vi "Controller server w pressure control.vi"() -> ()   [LabVIEW 2017]
uses:
  <vilib>/DAQmx/write.llb/DAQmx Write (Digital Bool 1Line 1Point).vi
  <vilib>/DAQmx/write.llb/DAQmx Write (Digital 1D Bool NChan 1Samp 1Line).vi
  <vilib>/DAQmx/read.llb/DAQmx Read (Digital 1D Bool NChan 1Samp 1Line).vi
  <vilib>/DAQmx/miscellaneous.llb/DAQmx Fill In Error Info.vi
panel:
  in  "Switch time (s)":dbl=20.0
  in  "Switch polarity":bool
  in  "Pressure control (psi)":dbl=40.0
  out "Gauge Pressure (psi)":dbl
  in  "Pressure controller":T1={"Unit ID"="A", "Baud Rate"=enum."19200", "VISA Sesssion In"="COM8"}
  in  "Potentiostat power":bool
  out "ALS START":bool
  in  "ALS START Contr.":bool
  in  "Valve 4 Contr.":bool
  out "HPLC pressure voltage":dbl format="%0.3f"
  out "ALS Ready":bool
  out "Valve 4":bool
  out "Pressure 2 (psi)":dbl
  in  "Pressure 2 calibrate":bool
  in  "50 psi voltage":dbl=1.184
  in  "200 psi voltage":dbl=3.211
  out "Pressure 2 voltage":dbl format="%0.3f"
  in  "A 3":dbl=74.00098667982239
  in  "B 3":dbl=-37.617168228909705
  out "Pressure 1 (psi)":dbl
  out "Pressure 1 voltage":dbl format="%0.3f"
  in  "Pressure 1 calibrate":bool
  in  "10 psi voltage":dbl=1.224
  in  "130 psi voltage":dbl=4.215
  in  "B 2":dbl=-39.1073219658977
  in  "A 2":dbl=40.120361083249755
  in  "0ml voltage":dbl=1.137
  in  "6ml voltage":dbl=3.445
  out "Position voltage":dbl format="%0.3f"
  in  "B 2":dbl=-2.9558058925476605
  in  "A 1":dbl=2.5996533795493937
  in  "Position calibrate":bool
  out "Pump 1 position":dbl format="%0.2f"
  in  "stop":bool
  in  "Manual control":bool
  out "HPLC pressure (bar)":dbl(graph)
  in  "Phase sensor calibrate":bool[](array[boolean])
  out "Phase sensor analog 6":dbl(graph)
  out "Phase sensor analog 5":dbl(graph)
  out "Valve 3":bool
  out "Valve 1 position":i32 max=1
  in  "Valve 3 Contr.":bool
  in  "Valve 2 Contr.":bool
  in  "Valve 1 Contr.":bool
  in  "HPLC SHUT DOWN Contr.":bool
  in  "HPLC START REQUEST Contr.":bool
  in  "HPLC STOP Contr.":bool
  in  "HPLC START Contr.":bool
  out "HPLC Ready":bool
  out "HPLC START REQUEST":bool
  out "HPLC STOP":bool
  out "HPLC SHUT DOWN":bool
  out "HPLC START":bool
  out "Phase sensor digital":bool[](array[boolean])
  out "Valve 1":bool
  out "Valve 2":bool
  out "Phase sensor analog 1":dbl(graph)
  out "Phase sensor analog 2":dbl(graph)
  out "Phase sensor analog 3":dbl(graph)
  out "Phase sensor analog 4":dbl(graph)
  # "Pressure transducer 1"
  # "Pressure transducer 2"
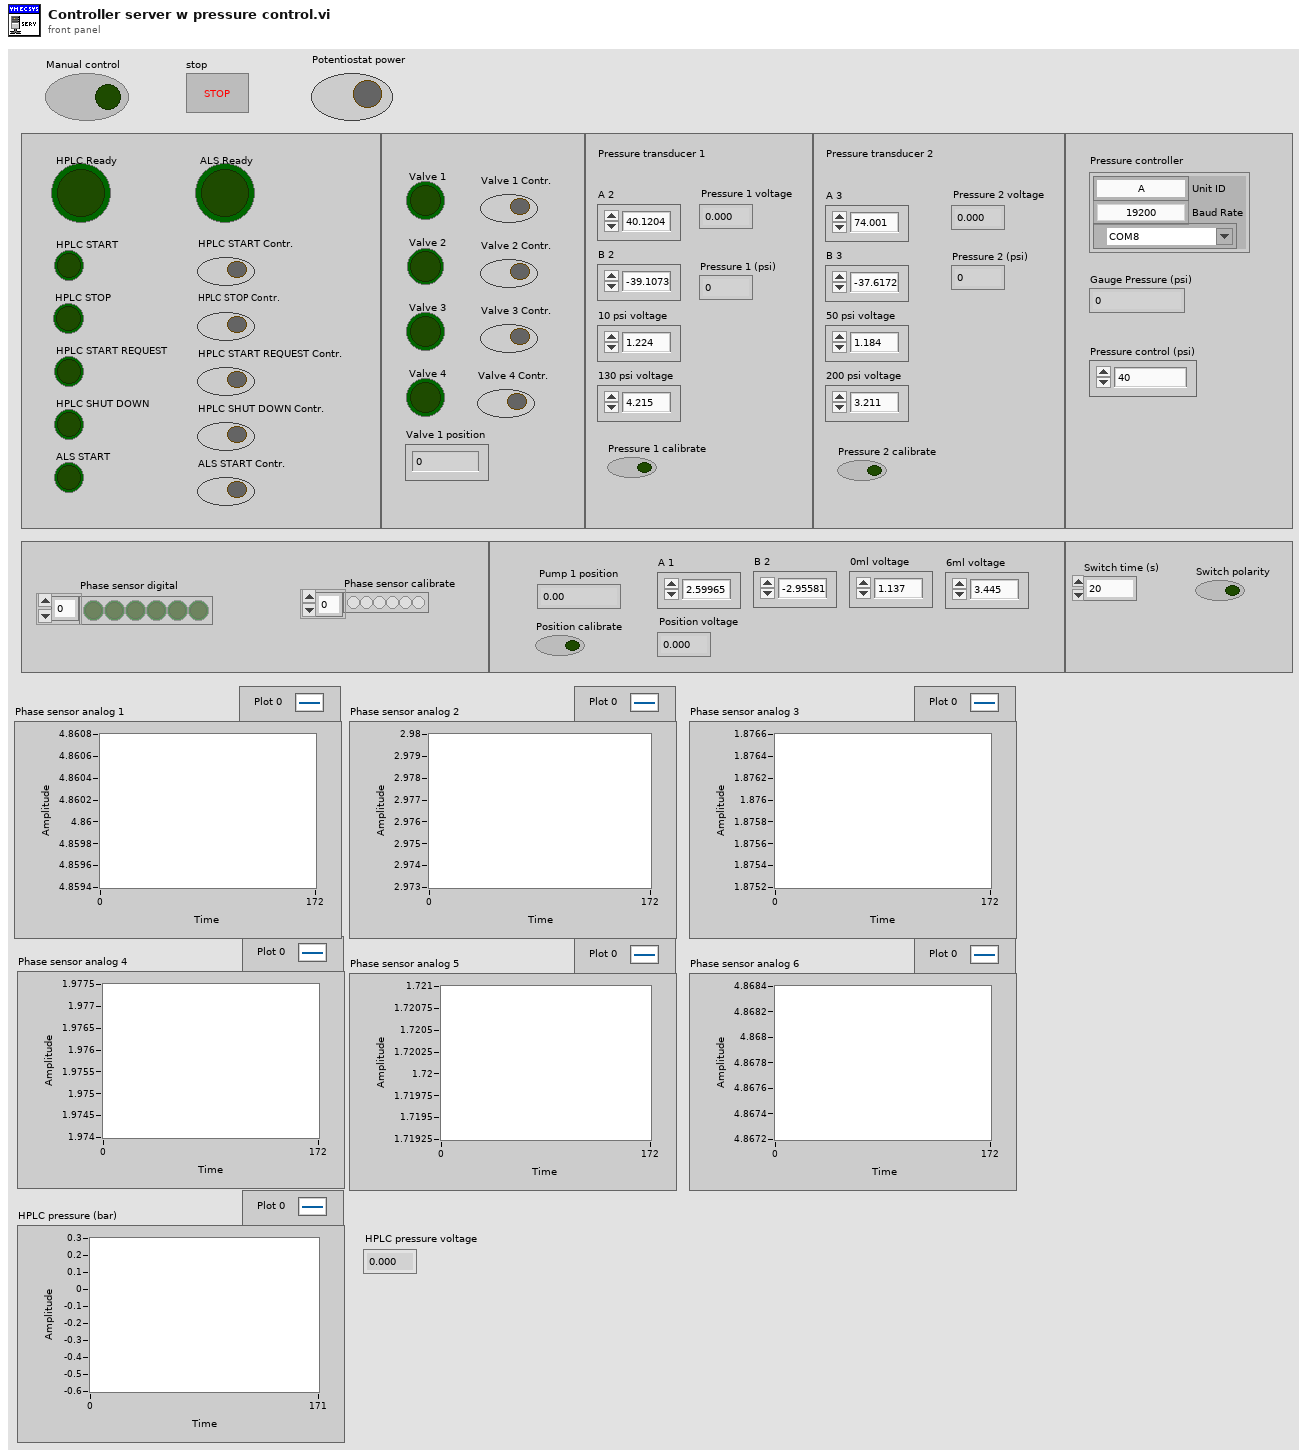
[diagram p1: front panel]
types:
  T1 = cluster{"Unit ID":string, "Baud Rate":enum8{"2400", "9600", "19200", "38400", "57600", "115200", "Unknown"}, "VISA Sesssion In":refnum<visa-resource-name>}
  T2 = cluster{"Absolute Pressure":bool, "Gauge/Diff. Pressure":bool, "Barometric Pressure":bool, "Temperature":bool, "Volumetric":bool, "Mass":bool, "Setpoint":bool, "Valve Drive":bool, "Totalizer":bool, "Totalizer Timer":bool, "Totalizer Average Flow":bool, "Totalizer Peak Flow":bool, "Gas Selected":bool, "Tot. Timer Format":u16}
  T3 = cluster{"Controller Full Scale":dbl, "Controller Select":u16, "Control Range":enum16{"Normal", "Inverted", "Bidirectional", "Unknown"}}
  T4 = cluster{"Absolute Pressure":dbl, "Gauge/Diff. Pressure":dbl, "Barometric Pressure":dbl, "Temperature":dbl, "Volumetric Flow":dbl, "Mass Flow":dbl, "Setpoint":dbl, "Valve Drive":dbl, "Totalizer":dbl, "[hr]":dbl, "[min]":dbl, "[sec]":dbl, "Totalizer Average Flow":dbl, "Totalizer Peak Flow":dbl, "Gas selected":string}
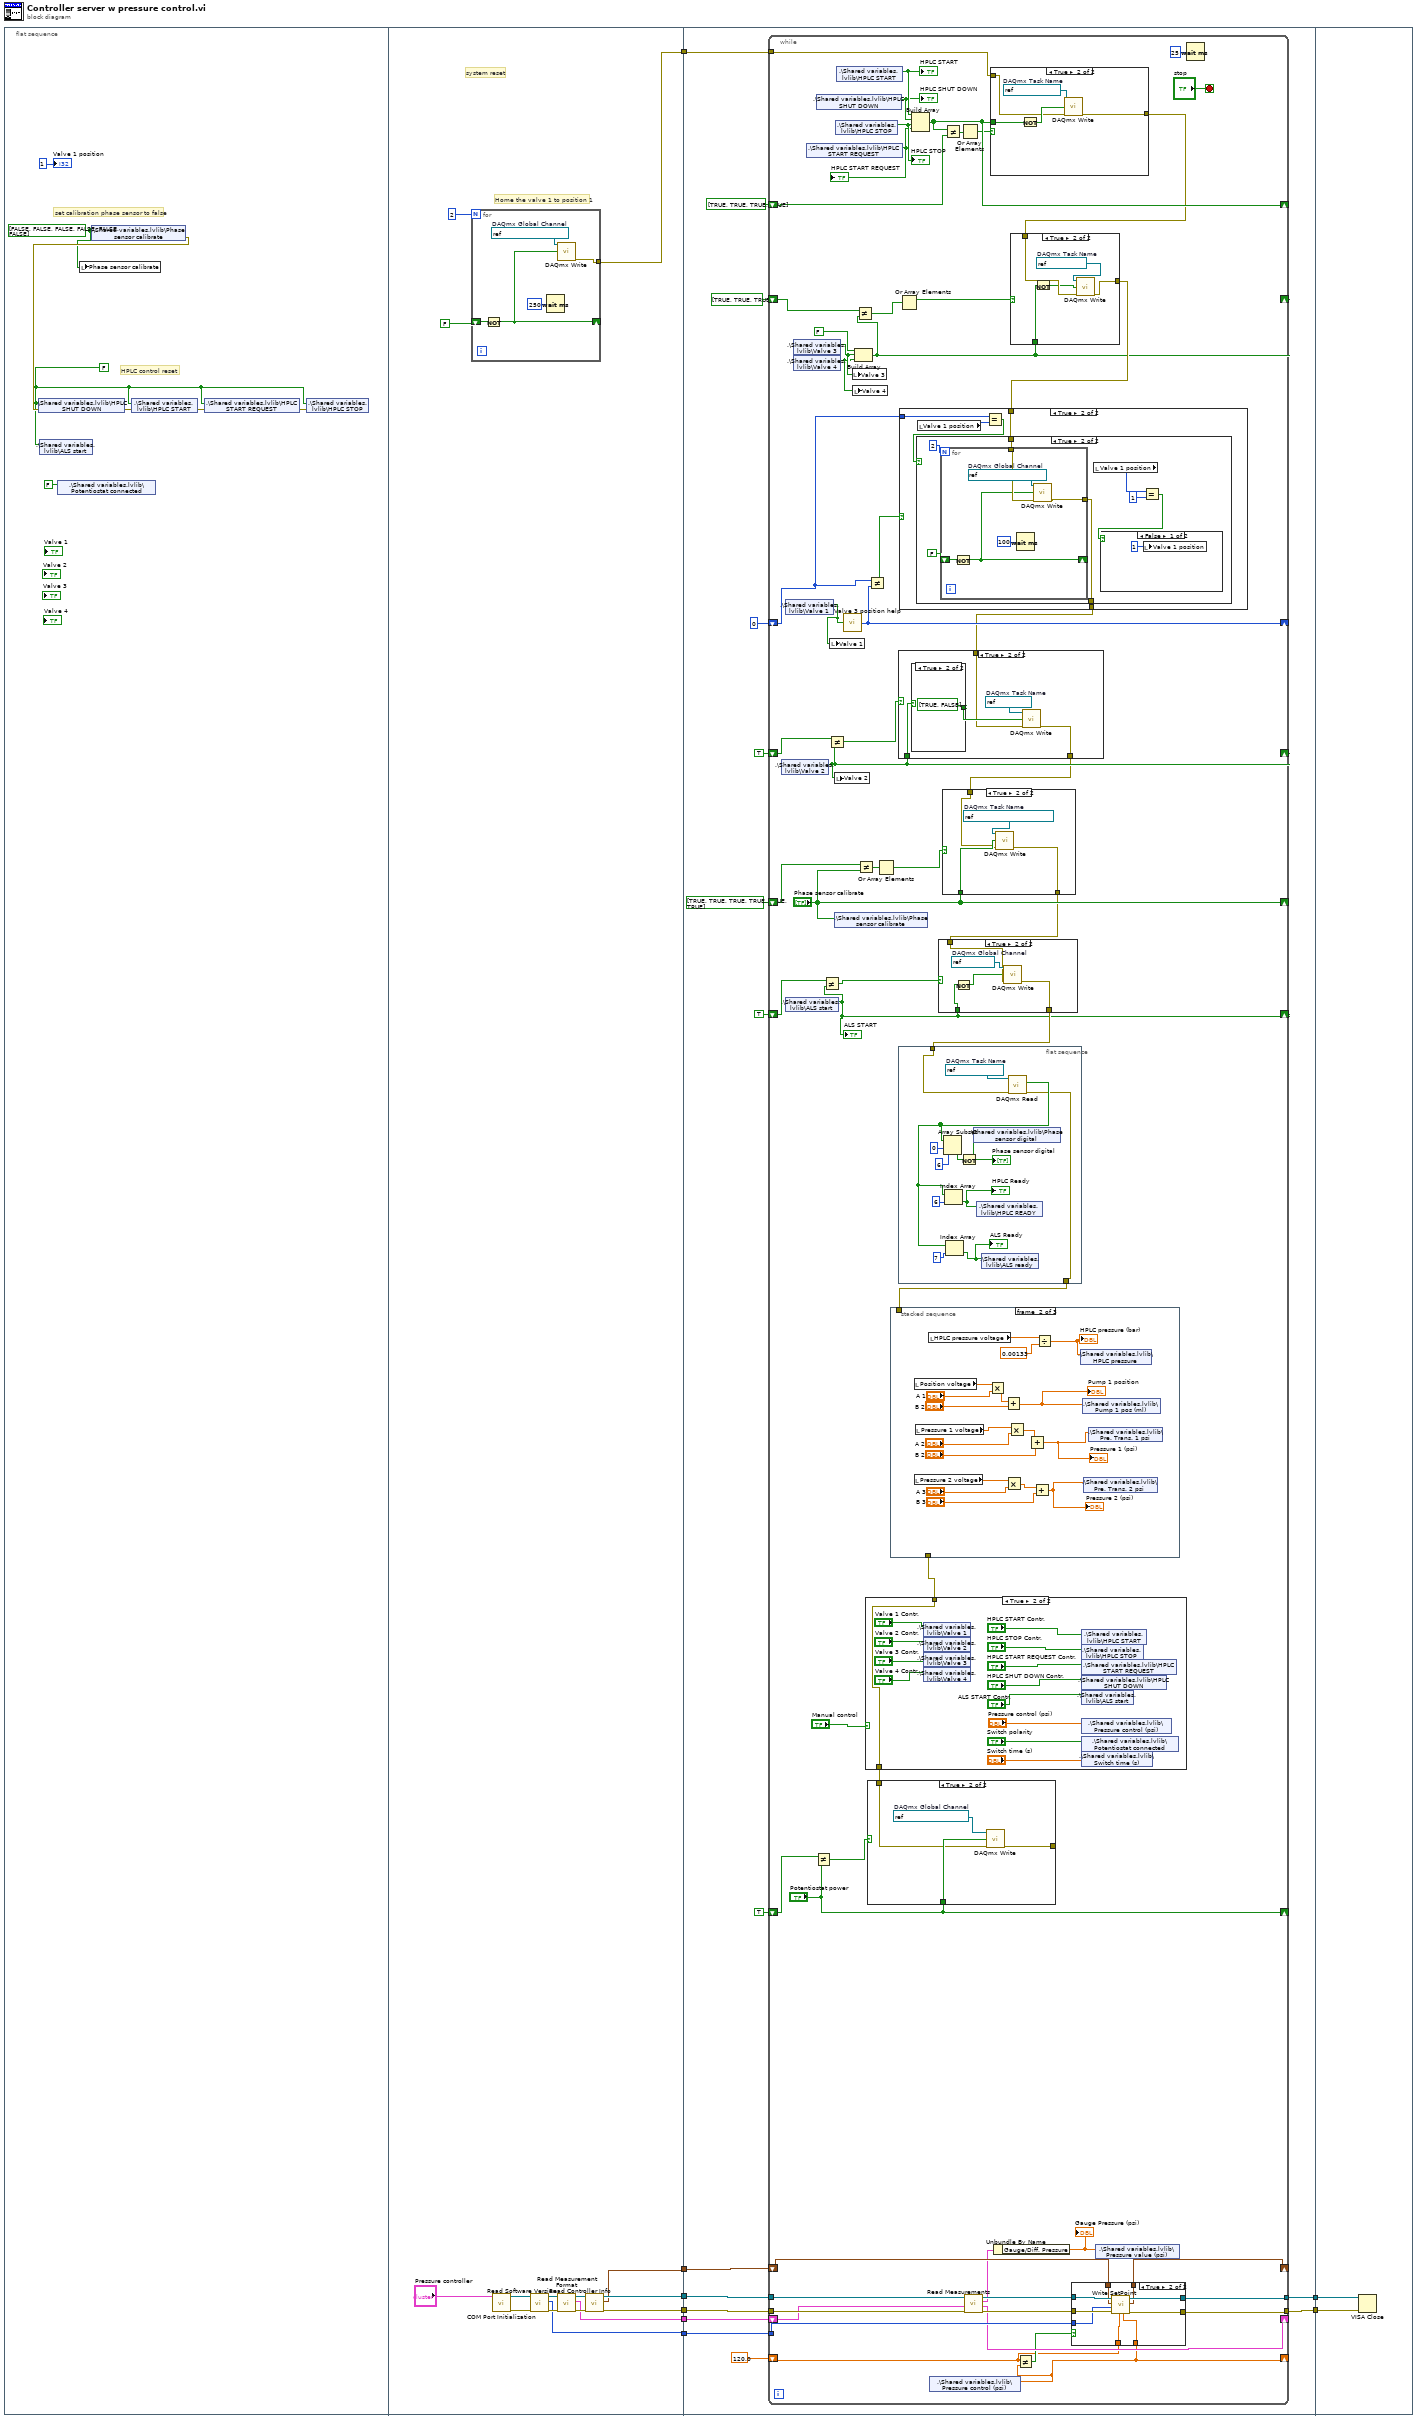
[diagram p0: block diagram]
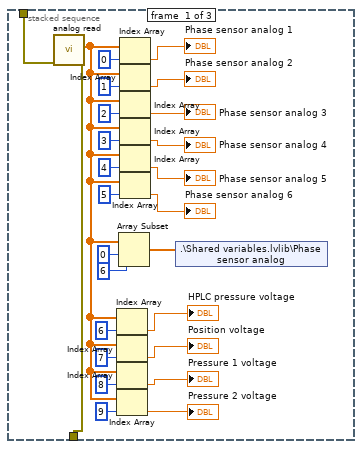
[diagram p4: hidden frame]
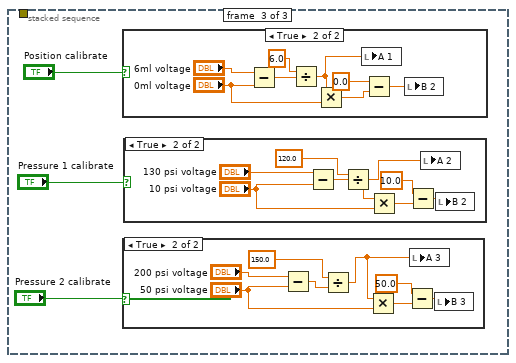
[diagram p5: hidden frame]
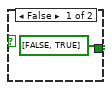
[diagram p11: hidden frame]
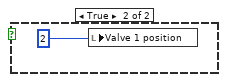
[diagram p16: hidden frame]
diagram:
  n1 = flat-sequence {
    tunnel: [w29] -> w8
    tunnel: [w21] -> w7
    tunnel: [w20] -> w6
    tunnel: [w19] -> w5
    tunnel: [w18] -> w4
    tunnel: [w17] -> w3
    tunnel: w8 -> [w51]
    tunnel: w7 -> [w45]
    tunnel: w6 -> [w44]
    tunnel: w5 -> [w43]
    tunnel: w4 -> [w42]
    tunnel: w3 -> [w41]
    tunnel: [w40] -> w2
    tunnel: [w39] -> w1
    tunnel: w2 -> [w282]
    tunnel: w1 -> [w281]
    frame #0 {
      w10 = FALSE
      w11 = bool[] [FALSE, FALSE, FALSE, FALSE, FALSE, FALSE] ("Phase sensor digital 2")
      # "HPLC control reset"
      # "set calibration phase sensor to false"
      n2 = shared-variable ".\\Shared variables.lvlib\\ALS start"(w10) -> ()  [unwired: 1 in, 1 out]
      n3 = shared-variable ".\\Shared variables.lvlib\\Potentiostat connected"(FALSE ("Switch polarity")) -> ()  [unwired: 1 in, 1 out]
      n4 = local write "Phase sensor calibrate"(w11) -> ()
      n5 = shared-variable ".\\Shared variables.lvlib\\Phase sensor calibrate"(w11) -> (error out=w16:errorcluster)  [unwired: 1 in]
      n6 = shared-variable ".\\Shared variables.lvlib\\HPLC SHUT DOWN"(w10, error in=w16) -> (error out=w15:errorcluster)
      n7 = shared-variable ".\\Shared variables.lvlib\\HPLC START"(w10, error in=w15) -> (error out=w14:errorcluster)
      n8 = shared-variable ".\\Shared variables.lvlib\\HPLC START REQUEST"(w10, error in=w14) -> (error out=w13:errorcluster)
      n9 = shared-variable ".\\Shared variables.lvlib\\HPLC STOP"(w10, error in=w13) -> ()  [unwired: 1 out]
      "Valve 1 position" <- 1 ("Valve 3 position")
    }
    frame #1 {
      # "Home the valve 1 to position 1"
      # "system reset"
      n10 = for {
        N: 2 -> [_]
        shift-right: [w32] -> _
        shift-left: FALSE -> [w36]
        tunnel: [w34] -> w29
        w33 = refnum<k21> "GILSON valve home"  # DAQmx Global Channel
        n11 = Not(x=w36) -> (.not. x?=w32:bool)
        n12 = Wait (ms)(milliseconds to wait=u32 250) -> ()  [unwired: 1 out]
        n13 = call-poly <vilib>:"DAQmx Write.vi"("task/channels in"=w33, "data"=w32) -> ("error out"=w34:errorcluster)  [unwired: 11 in, 2 out]
      }
      n14 = call <instrlib>:"COM Port Initialization.vi"("Communication Settings"="Pressure controller") -> ("error out"=w23:errorcluster, "VISA Session Out"=w24:refnum<visa-resource-name>)  [unwired: 9 in]
      n15 = call <instrlib>:"Read Software Version.vi"("error in"=w23, "VISA Session In"=w24) -> ("error out"=w28:errorcluster, "Software Version"=w17:u8, "VISA Session Out"=w27:refnum<visa-resource-name>)  [unwired: 7 in]
      n16 = call <instrlib>:"Read Measurement Format.vi"("error in"=w28, "VISA Session In"=w27) -> ("error out"=w26:errorcluster, "Data Frame Format"=w18:T2, "VISA Session Out"=w25:refnum<visa-resource-name>)  [unwired: 7 in]
      n17 = call <instrlib>:"Read Controller Info.vi"("error in"=w26, "VISA Session In"=w25) -> ("error out"=w20:errorcluster, "Controller Info out"=w19:T3, "VISA Session Out"=w21:refnum<visa-resource-name>)  [unwired: 6 in, 1 out]
    }
    frame #2 {
      n18 = while {
        shift-right: [w92] -> _
        shift-left: bool[] [TRUE, TRUE, TRUE] -> [w93]
        shift-right: [w107] -> _
        shift-left: bool[] [TRUE, TRUE, TRUE, TRUE] ("Phase sensor digital 2") -> [w108]
        tunnel: w51 -> [w104]
        shift-right: [w89] -> _
        shift-left: 0 ("Numeric") -> [w88]
        shift-right: ["Phase sensor calibrate"] -> _
        shift-left: bool[] [TRUE, TRUE, TRUE, TRUE, TRUE, TRUE] ("Phase sensor calibrate") -> [w81]
        shift-right: [w85] -> _
        shift-left: TRUE ("Boolean") -> [w86]
        shift-right: [w73] -> _
        shift-left: TRUE ("Boolean") -> [w79]
        shift-right: ["Potentiostat power"] -> _
        shift-left: TRUE ("Potentiostat power") -> [w71]
        shift-right: [w61] -> _
        shift-left: w43 -> [w63]
        shift-right: [w60] -> _
        shift-left: w42 -> [w62]
        shift-right: [w58] -> _
        shift-left: 120.0 ("Double") -> [w57]
        tunnel: w45 -> [w66]
        tunnel: w44 -> [w65]
        tunnel: w41 -> [w64]
        tunnel: [w56] -> w40
        tunnel: [w55] -> w39
        stop <- "stop" stop-if-true
        n19 = shared-variable ".\\Shared variables.lvlib\\Valve 2"() -> (w85:bool)  [unwired: 1 in, 1 out]
        n20 = shared-variable ".\\Shared variables.lvlib\\ALS start"() -> (w73:bool)  [unwired: 1 in, 1 out]
        "ALS START" <- w73
        n21 = shared-variable ".\\Shared variables.lvlib\\Valve 1"() -> (w87:bool)  [unwired: 1 in, 1 out]
        n22 = shared-variable ".\\Shared variables.lvlib\\Valve 3"() -> (w91:bool)  [unwired: 1 in, 1 out]
        n23 = shared-variable ".\\Shared variables.lvlib\\Valve 4"() -> (w90:bool)  [unwired: 1 in, 1 out]
        n24 = shared-variable ".\\Shared variables.lvlib\\HPLC START REQUEST"() -> (w109:bool)  [unwired: 1 in, 1 out]
        "HPLC START REQUEST" <- w109
        n25 = Not Equal?(x=w71, y="Potentiostat power") -> (x != y?=w72:bool)
        n26 = shared-variable ".\\Shared variables.lvlib\\HPLC SHUT DOWN"() -> (w111:bool)  [unwired: 1 in, 1 out]
        "HPLC SHUT DOWN" <- w111
        n27 = Not Equal?(x=w79, y=w73) -> (x != y?=w78:bool)
        n28 = Not Equal?(x=w86, y=w85) -> (x != y?=w84:bool)
        n29 = local write "Valve 1"(w87) -> ()
        n30 = local write "Valve 2"(w85) -> ()
        n31 = shared-variable ".\\Shared variables.lvlib\\Phase sensor calibrate"("Phase sensor calibrate") -> ()  [unwired: 1 in, 1 out]
        n32 = shared-variable ".\\Shared variables.lvlib\\HPLC STOP"() -> (w110:bool)  [unwired: 1 in, 1 out]
        "HPLC STOP" <- w110
        n33 = shared-variable ".\\Shared variables.lvlib\\HPLC START"() -> (w112:bool)  [unwired: 1 in, 1 out]
        "HPLC START" <- w112
        n34 = call "Valve 3 position help.vi"("Boolean"=w87) -> ("Numeric"=w89:i32)
        n35 = local write "Valve 3"(w91) -> ()
        n36 = local write "Valve 4"(w90) -> ()
        n37 = Build Array(FALSE ("element"), w91, w90) -> (w92:bool[])
        n38 = Not Equal?(x=w93, y=w92) -> (x != y?=w95:bool[])
        n39 = Not Equal?(x=w81, y="Phase sensor calibrate") -> (x != y?=w102:bool[])
        n40 = Not Equal?(x=w88, y=w89) -> (x != y?=w103:bool)
        n41 = Or Array Elements(Boolean array=w102) -> (logical OR=w101:bool)
        n42 = stacked-sequence {
          tunnel: w75 -> [w141 _ _]
          tunnel: [w135 _ _] -> w74
          frame #0 {
            n43 = call "analog read.vi"("error in"=w141) -> ("error out"=w135:errorcluster, "data"=w140:dbl[])  [unwired: 9 in]
            n44 = Index Array(array=w140, index=6) -> (element=→"HPLC pressure voltage":dbl)
            n45 = Index Array(array=w140, index=7) -> (element=→"Position voltage":dbl)
            n46 = Index Array(array=w140, index=8) -> (element=→"Pressure 1 voltage":dbl)
            n47 = Index Array(array=w140, index=9) -> (element=→"Pressure 2 voltage":dbl)
            n48 = Array Subset(array=w140, index=0, length=6) -> (w142:dbl[])
            n49 = Index Array(array=w140, index=0) -> (element=→"Phase sensor analog 1":dbl)
            n50 = Index Array(array=w140, index=1) -> (element=→"Phase sensor analog 2":dbl)
            n51 = Index Array(array=w140, index=2) -> (element=→"Phase sensor analog 3":dbl)
            n52 = Index Array(array=w140, index=3) -> (element=→"Phase sensor analog 4":dbl)
            n53 = Index Array(array=w140, index=4) -> (element=→"Phase sensor analog 5":dbl)
            n54 = Index Array(array=w140, index=5) -> (element=→"Phase sensor analog 6":dbl)
            n55 = shared-variable ".\\Shared variables.lvlib\\Phase sensor analog"(w142) -> ()  [unwired: 1 in, 1 out]
          }
          frame #1 {
            n56 = local read "Position voltage"() -> (w167:dbl)
            n57 = local read "Pressure 2 voltage"() -> (w157:dbl)
            n58 = local read "Pressure 1 voltage"() -> (w163:dbl)
            n59 = local read "HPLC pressure voltage"() -> (w172:dbl)
            n60 = Multiply(x=w167, y="A 1") -> (x*y=w170:dbl)
            n61 = Add(x=w170, y="B 2") -> (x+y=w171:dbl)
            "Pump 1 position" <- w171
            n62 = Multiply(x=w157, y="A 3") -> (x*y=w159:dbl)
            n63 = Multiply(x=w163, y="A 2") -> (x*y=w162:dbl)
            n64 = Add(x=w162, y="B 2") -> (x+y=w166:dbl)
            "Pressure 1 (psi)" <- w166
            n65 = Add(x=w159, y="B 3") -> (x+y=w161:dbl)
            "Pressure 2 (psi)" <- w161
            n66 = Divide(x=w172, y=0.00133) -> (x/y=w174:dbl)
            "HPLC pressure (bar)" <- w174
            n67 = shared-variable ".\\Shared variables.lvlib\\HPLC pressure"(w174) -> ()  [unwired: 1 in, 1 out]
            n68 = shared-variable ".\\Shared variables.lvlib\\Pump 1 pos (ml)"(w171) -> ()  [unwired: 1 in, 1 out]
            n69 = shared-variable ".\\Shared variables.lvlib\\Pre. Trans. 2 psi"(w161) -> ()  [unwired: 1 in, 1 out]
            n70 = shared-variable ".\\Shared variables.lvlib\\Pre. Trans. 1 psi"(w166) -> ()  [unwired: 1 in, 1 out]
          }
          frame #2 {
            n71 = case shown="True" "Position calibrate" {
              frame False {
              }
              frame True {
                n72 = Subtract(x="6ml voltage", y="0ml voltage") -> (x-y=w194:dbl)
                n73 = Divide(x=6.0 ("y"), y=w194) -> (x/y=w200:dbl)
                n74 = Multiply(x=w200, y="0ml voltage") -> (x*y=w198:dbl)
                n75 = local write "A 1"(w200) -> ()
                n76 = Subtract(x=0.0, y=w198) -> (x-y=w196:dbl)
                n77 = local write "B 2"(w196) -> ()
              }
            }
            n78 = case shown="True" "Pressure 2 calibrate" {
              frame False {
              }
              frame True {
                n79 = Subtract(x="200 psi voltage", y="50 psi voltage") -> (x-y=w180:dbl)
                n80 = Divide(x=150.0 ("y"), y=w180) -> (x/y=w185:dbl)
                n81 = Multiply(x=w185, y="50 psi voltage") -> (x*y=w184:dbl)
                n82 = Subtract(x=50.0, y=w184) -> (x-y=w182:dbl)
                n83 = local write "A 3"(w185) -> ()
                n84 = local write "B 3"(w182) -> ()
              }
            }
            n85 = case shown="True" "Pressure 1 calibrate" {
              frame False {
              }
              frame True {
                n86 = Subtract(x="130 psi voltage", y="10 psi voltage") -> (x-y=w188:dbl)
                n87 = Divide(x=120.0 ("y"), y=w188) -> (x/y=w193:dbl)
                n88 = Multiply(x=w193, y="10 psi voltage") -> (x*y=w192:dbl)
                n89 = Subtract(x=10.0, y=w192) -> (x-y=w190:dbl)
                n90 = local write "A 2"(w193) -> ()
                n91 = local write "B 2"(w190) -> ()
              }
            }
          }
        }
        n92 = case shown="True" "Manual control" {
          tunnel: w74 -> [w228 w232]
          tunnel: [w228 w232] -> w69
          frame False {
          }
          frame True {
            n93 = shared-variable ".\\Shared variables.lvlib\\Valve 1"("Valve 1 Contr.") -> ()  [unwired: 1 in, 1 out]
            n94 = shared-variable ".\\Shared variables.lvlib\\Valve 2"("Valve 2 Contr.") -> ()  [unwired: 1 in, 1 out]
            n95 = shared-variable ".\\Shared variables.lvlib\\Valve 3"("Valve 3 Contr.") -> ()  [unwired: 1 in, 1 out]
            n96 = shared-variable ".\\Shared variables.lvlib\\Valve 4"("Valve 4 Contr.") -> ()  [unwired: 1 in, 1 out]
            n97 = shared-variable ".\\Shared variables.lvlib\\HPLC START"("HPLC START Contr.") -> ()  [unwired: 1 in, 1 out]
            n98 = shared-variable ".\\Shared variables.lvlib\\HPLC STOP"("HPLC STOP Contr.") -> ()  [unwired: 1 in, 1 out]
            n99 = shared-variable ".\\Shared variables.lvlib\\HPLC START REQUEST"("HPLC START REQUEST Contr.") -> ()  [unwired: 1 in, 1 out]
            n100 = shared-variable ".\\Shared variables.lvlib\\HPLC SHUT DOWN"("HPLC SHUT DOWN Contr.") -> ()  [unwired: 1 in, 1 out]
            n101 = shared-variable ".\\Shared variables.lvlib\\ALS start"("ALS START Contr.") -> ()  [unwired: 1 in, 1 out]
            n102 = shared-variable ".\\Shared variables.lvlib\\Pressure control (psi)"("Pressure control (psi)") -> ()  [unwired: 1 in, 1 out]
            n103 = shared-variable ".\\Shared variables.lvlib\\Potentiostat connected"("Switch polarity") -> ()  [unwired: 1 in, 1 out]
            n104 = shared-variable ".\\Shared variables.lvlib\\Switch time (s)"("Switch time (s)") -> ()  [unwired: 1 in, 1 out]
          }
        }
        n105 = case shown="True" w72 {
          tunnel: "Potentiostat power" -> [_ w129]
          tunnel: w69 -> [w126 w128]
          tunnel: [w126 w127] -> _
          frame False {
          }
          frame True {
            w130 = refnum<k21> "Potentiostat power"  # DAQmx Global Channel
            n106 = call-poly <vilib>:"DAQmx Write.vi"("task/channels in"=w130, "data"=w129, "error in"=w128) -> ("error out"=w127:errorcluster)  [unwired: 10 in, 2 out]
          }
        }
        n107 = flat-sequence {
          tunnel: w76 -> [w206]
          tunnel: [w202] -> w75
          frame #0 {
            w210 = refnum<k21> "system status"  # DAQmx Task Name
            n108 = call-poly <vilib>:"DAQmx Read.vi"("task/channels in"=w210, "error in"=w206) -> ("data"=w204:bool[], "error out"=w202:errorcluster)  [unwired: 11 in, 1 out]
            n109 = Array Subset(array=w204, index=0, length=6) -> (w208:bool[])
            n110 = Index Array(array=w204, index=6) -> (element=w209:bool)
            "HPLC Ready" <- w209
            n111 = Index Array(array=w204, index=7) -> (element=w203:bool)
            "ALS Ready" <- w203
            n112 = Not(x=w208) -> (.not. x?=w207:bool[])
            "Phase sensor digital" <- w207
            n113 = shared-variable ".\\Shared variables.lvlib\\Phase sensor digital"(w207) -> ()  [unwired: 1 in, 1 out]
            n114 = shared-variable ".\\Shared variables.lvlib\\HPLC READY"(w209) -> ()  [unwired: 1 in, 1 out]
            n115 = shared-variable ".\\Shared variables.lvlib\\ALS ready"(w203) -> ()  [unwired: 1 in, 1 out]
          }
        }
        n116 = Or Array Elements(Boolean array=w95) -> (logical OR=w113:bool)
        n117 = Build Array(w112, w111, w110, w109) -> (w107:bool[])
        n118 = shared-variable ".\\Shared variables.lvlib\\Pressure control (psi)"() -> (w58:dbl)  [unwired: 1 in, 1 out]
        n119 = Not Equal?(x=w107, y=w108) -> (x != y?=w106:bool[])
        n120 = Or Array Elements(Boolean array=w106) -> (logical OR=w105:bool)
        n121 = call <instrlib>:"Read Measurements.vi"("error in"=w65, "Data Frame Format In"=w62, "VISA Session In"=w66) -> ("error out"=w67:errorcluster, "Data Frame Format Out"=w60:T2, "Data Cluster"=w53:T4, "VISA Session Out"=w68:refnum<visa-resource-name>)  [unwired: 1 in, 4 out]
        n122 = case shown="True" w105 {
          tunnel: w107 -> [_ w274]
          tunnel: [w269 w272] -> w97
          tunnel: w104 -> [w269 w271]
          frame False {
          }
          frame True {
            w270 = refnum<k21> "HPLC control"  # DAQmx Task Name
            n123 = Not(x=w274) -> (.not. x?=w273:bool[])
            n124 = call-poly <vilib>:"DAQmx Write.vi"("task/channels in"=w270, "data"=w273, "error in"=w271) -> ("error out"=w272:errorcluster)  [unwired: 10 in, 2 out]
          }
        }
        n125 = Unbundle By Name(w53) -> ("Gauge/Diff. Pressure"=w54:dbl)
        "Gauge Pressure (psi)" <- w54
        n126 = case shown="True" w113 {
          tunnel: w97 -> [w275 w279]
          tunnel: [w275 w278] -> w98
          tunnel: w92 -> [_ w276]
          frame False {
          }
          frame True {
            w280 = refnum<k21> "IDEX valves"  # DAQmx Task Name
            n127 = Not(x=w276) -> (.not. x?=w277:bool[])
            n128 = call-poly <vilib>:"DAQmx Write.vi"("task/channels in"=w280, "data"=w277, "error in"=w279) -> ("error out"=w278:errorcluster)  [unwired: 10 in, 2 out]
          }
        }
        n129 = case shown="True" w103 {
          tunnel: w88 -> [_ w251]
          tunnel: w98 -> [w247 w249]
          tunnel: [w247 w248] -> w83
          frame False {
          }
          frame True {
            n130 = local read "Valve 1 position"() -> (w252:i32)
            n131 = Equal?(x=w251, y=w252) -> (x = y?=w250:bool)
            n132 = case shown="True" w250 {
              tunnel: w249 -> [w253 w255]
              tunnel: [w253 w254] -> w248
              frame False {
              }
              frame True {
                n133 = for {
                  N: 2 -> [_]
                  shift-right: [w263] -> _
                  shift-left: FALSE -> [w268]
                  tunnel: w255 -> [w265]
                  tunnel: [w266] -> w254
                  w264 = refnum<k21> "GILSON valve switch"  # DAQmx Global Channel
                  n134 = Not(x=w268) -> (.not. x?=w263:bool)
                  n135 = Wait (ms)(milliseconds to wait=u32 100) -> ()  [unwired: 1 out]
                  n136 = call-poly <vilib>:"DAQmx Write.vi"("task/channels in"=w264, "data"=w263, "error in"=w265) -> ("error out"=w266:errorcluster)  [unwired: 10 in, 2 out]
                }
                n137 = local read "Valve 1 position"() -> (w258:i32)
                n138 = Equal?(x=w258, y=1) -> (x = y?=w256:bool)
                n139 = case shown="False" w256 {
                  frame False {
                    n140 = local write "Valve 1 position"(1 ("Valve 3 position")) -> ()
                  }
                  frame True {
                    n141 = local write "Valve 1 position"(2 ("y")) -> ()
                  }
                }
              }
            }
          }
        }
        n142 = case shown="True" w84 {
          tunnel: w85 -> [_ w225]
          tunnel: w83 -> [w220 w222]
          tunnel: [w220 w221] -> w82
          frame False {
          }
          frame True {
            w224 = refnum<k21> "VICI valve"  # DAQmx Task Name
            n143 = case shown="True" w225 {
              tunnel: [bool[] [FALSE, TRUE] ("data") bool[] [TRUE, FALSE] ("data")] -> w223
              frame False {
              }
              frame True {
              }
            }
            n144 = call-poly <vilib>:"DAQmx Write.vi"("task/channels in"=w224, "data"=w223, "error in"=w222) -> ("error out"=w221:errorcluster)  [unwired: 10 in, 2 out]
          }
        }
        n145 = case shown="True" w101 {
          tunnel: "Phase sensor calibrate" -> [_ w246]
          tunnel: [w242 w244] -> w77
          tunnel: w82 -> [w242 w243]
          frame False {
          }
          frame True {
            w245 = refnum<k21> "Phase sensor calibration"  # DAQmx Task Name
            n146 = call-poly <vilib>:"DAQmx Write.vi"("task/channels in"=w245, "data"=w246, "error in"=w243) -> ("error out"=w244:errorcluster)  [unwired: 10 in, 2 out]
          }
        }
        n147 = case shown="True" w78 {
          tunnel: w73 -> [_ w215]
          tunnel: w77 -> [w214 w218]
          tunnel: [w214 w217] -> w76
          frame False {
          }
          frame True {
            w219 = refnum<k21> "ALS start"  # DAQmx Global Channel
            n148 = Not(x=w215) -> (.not. x?=w216:bool)
            n149 = call-poly <vilib>:"DAQmx Write.vi"("task/channels in"=w219, "data"=w216, "error in"=w218) -> ("error out"=w217:errorcluster)  [unwired: 10 in, 2 out]
          }
        }
        n150 = Not Equal?(x=w57, y=w58) -> (x != y?=w59:bool)
        n151 = case shown="True" w59 {
          tunnel: w68 -> [w116 w125]
          tunnel: w67 -> [w115 w124]
          tunnel: [w115 w123] -> w55
          tunnel: [w116 w122] -> w56
          tunnel: [w114 w121] -> w61
          tunnel: w64 -> [_ w120]
          tunnel: w63 -> [w114 w119]
          tunnel: w58 -> [_ w118]
          tunnel: w57 -> [_ w117]
          frame False {
          }
          frame True {
            n152 = call <instrlib>:"Write SetPoint.vi"("Setpoint"=w118, "Previous Setpoint"=w117, "error in"=w124, "Software Version"=w120, "Controller Info out"=w119, "VISA Session In"=w125) -> ("error out"=w123:errorcluster, "Controller Info out"=w121:T3, "VISA Session Out"=w122:refnum<visa-resource-name>)  [unwired: 2 in, 1 out]
          }
        }
        n153 = shared-variable ".\\Shared variables.lvlib\\Pressure value (psi)"(w54) -> ()  [unwired: 1 in, 1 out]
        n154 = Wait (ms)(milliseconds to wait=u32 25) -> ()  [unwired: 1 out]
      }
    }
    frame #3 {
      n155 = VISA Close(VISA resource name=w282, error in (no error)=w281) -> ()  [unwired: 1 out]
    }
  }
